vi "Decimal to 2sComp.vi"(10 "size in bit":u8=9, 11 "decimal in":dbl) -> (3 "word out":dbl=2057.0 format="%.2f")   [LabVIEW 2020, in "dt_encodeDecode.lvlib"]
uses:
  dt_encodeDecode.lvlib
panel:
  out "int 2":u32=2057 format="%.0b"
  out "int 1":u32=2057 format="%.0b"
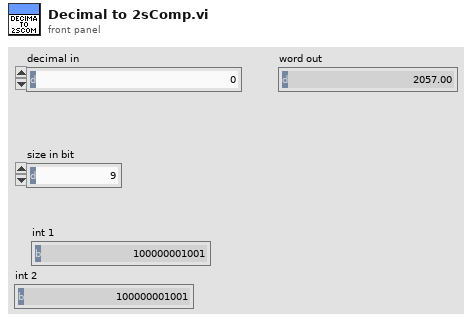
[diagram p1: front panel]
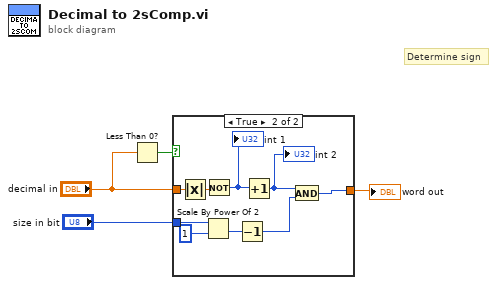
[diagram p0: block diagram]
diagram:
  # "Determine sign"
  n1 = Less Than 0?(x="decimal in") -> (x < 0?=w2:bool)
  n2 = case shown="True" w2 {
    tunnel: [w5 w10] -> w4
    tunnel: "decimal in" -> [w5 w14]
    tunnel: "size in bit" -> [_ w13]
    frame False {
    }
    frame True {
      n3 = Absolute Value(x=w14) -> (abs(x)=w6:dbl)
      n4 = Scale By Power Of 2(n=w13, x=1) -> (x*2^n=w11:i32)
      n5 = Not(x=w6) -> (.not. x?=w8:u32)
      "int 1" <- w8
      n6 = Decrement(x=w11) -> (x-1=w9:i32)
      n7 = Increment(x=w8) -> (x+1=w7:u32)
      "int 2" <- w7
      n8 = And(x=w7, y=w9) -> (x .and. y?=w10:u32)
    }
  }
  "word out" <- w4
